vi "b(perm).vi"(4 "Label":dbl[](array[numeric]), 5 "tol":dbl, 6 "nin":dbl, 7 "Q":T1, 8 "Boolean":bool, 9 "Rank":i16, 10 "P":i32[][](array[numeric]), 11 "R":T1) -> (0 "perm":i32[](array[numeric]), 1 "b(perm)":dbl[](array[numeric]), 2 "Q":T1, 3 "R":T1)   [LabVIEW 2014]
uses:
  <vilib>/Analysis/Matrix/Datatypes/RealMatrix.ctl
  <vilib>/Analysis/baseanly.llb/A x Vector.vi
  <vilib>/Analysis/baseanly.llb/Real Inverse Matrix.vi
  <vilib>/Analysis/NI_AALBase.lvlib
  <vilib>/Analysis/Matrix/NI_Matrix.lvlib
panel:
  # "INPUTS"
  # "OUTPUTS"
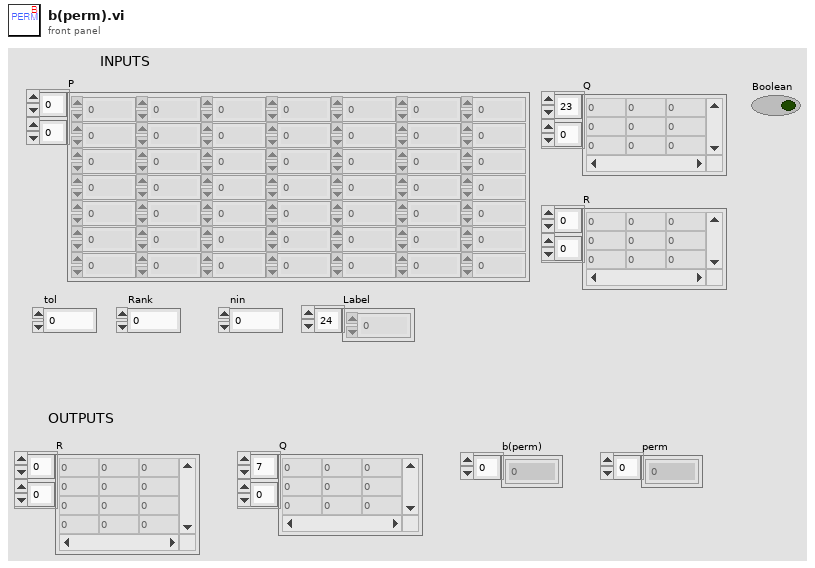
[diagram p1: front panel]
types:
  T1 = typedef "NI_Matrix.lvlib/RealMatrix.ctl" = dbl[][]
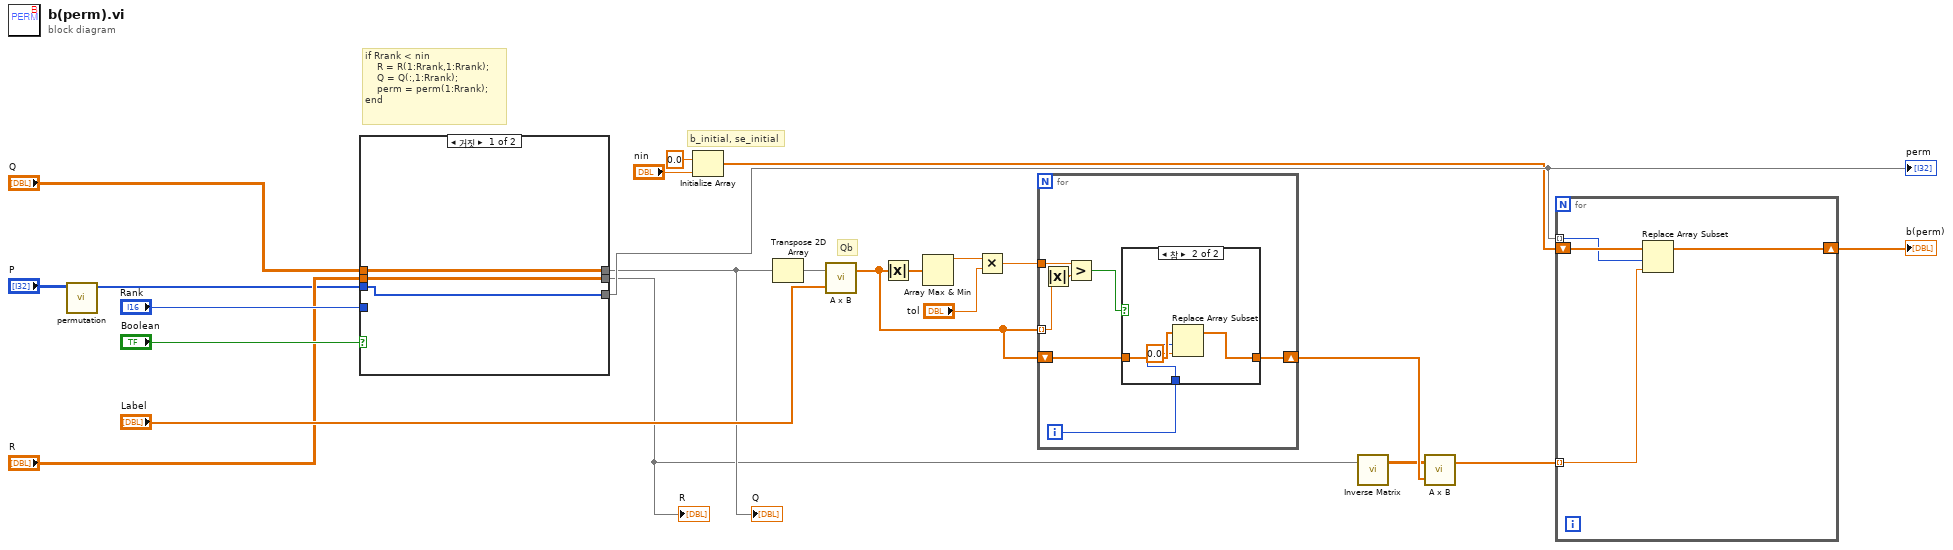
[diagram p0: block diagram]
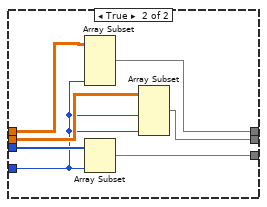
[diagram p3: hidden frame]
diagram:
  # "Qb"
  # "b_initial, se_initial"
  # "if Rrank < nin\n    R = R(1:Rrank,1:Rrank);\n    Q = Q(:,1:Rrank);\n    perm = perm(1:Rrank);\nend"
  n1 = call "permutation.vi"("P"="P") -> ("permutation"=w5:i32[])  [unwired: 10 in]
  n2 = case shown="거짓" "Boolean" {
    tunnel: "R" -> [w25 w29]
    tunnel: "Q" -> [w26 w31]
    tunnel: w5 -> [w24 w33]
    tunnel: "Rank" -> [_ w27]
    tunnel: [w26 w30] -> w6
    tunnel: [w25 w28] -> w1
    tunnel: [w24 w32] -> w23
    frame False {
    }
    frame True {
      n3 = Array Subset(array=w31, length (col)=w27) -> (w30:T1)  [unwired: 3 in]
      n4 = Array Subset(array=w33, length=w27) -> (w32:i32[])  [unwired: 1 in]
      n5 = Array Subset(array=w29, length (row)=w27, length (col)=w27) -> (w28:T1)  [unwired: 2 in]
    }
  }
  "R" <- w1
  "Q" <- w6
  "perm" <- w23
  n6 = Initialize Array(0.0 ("element"), "nin") -> (w9:dbl[])
  n7 = Transpose 2D Array(2D array=w6) -> (transposed array=w3:T1)
  n8 = call-poly <vilib>:"A x B.vi"("Vector"="Label", "A"=w3) -> ("A x Vector"=w19:dbl[])  [unwired: 1 out]
  n9 = Absolute Value(x=w19) -> (abs(x)=w2:dbl[])
  n10 = Array Max & Min(array=w2) -> (max value=w16:dbl)  [unwired: 3 out]
  n11 = Multiply(x=w16, y="tol") -> (x*y=w18:dbl)
  n12 = for {
    tunnel: w19 -> [w39] mode=indexing
    tunnel: w18 -> [w40]
    shift-right: [w36] -> w21
    shift-left: w19 -> [w35]
    i -> [w37]
    n13 = Absolute Value(x=w39) -> (abs(x)=w34:dbl)
    n14 = Greater?(x=w40, y=w34) -> (0:w38:bool)
    n15 = case shown="참" w38 {
      tunnel: w35 -> [w41 w45]
      tunnel: w37 -> [_ w44]
      tunnel: [w41 w42] -> w36
      frame False {
      }
      frame True {
        n16 = Replace Array Subset(array=w45, new element=0.0 ("new element/subarray"), index=w44) -> (w42:dbl[])
      }
    }
  }
  n17 = call-poly <vilib>:"Inverse Matrix.vi"("Input Matrix"=w1) -> ("Inverse Matrix"=w20:T1)  [unwired: 1 in, 1 out]
  n18 = call-poly <vilib>:"A x B.vi"("Vector"=w21, "A"=w20) -> ("A x Vector"=w22:dbl[])  [unwired: 1 out]
  n19 = for {
    tunnel: w22 -> [w49] mode=indexing
    tunnel: w23 -> [w46] mode=indexing
    shift-right: [w48] -> w4
    shift-left: w9 -> [w47]
    n20 = Replace Array Subset(array=w47, new element=w49, index=w46) -> (w48:dbl[])
  }
  "b(perm)" <- w4
